vi "Set Scan Settings.vi"(10 "Test Settings":T1 {"Load Cell Sensitivity" format="%.6f"}, 11 "Model in":refnum<class "Model.lvclass">) -> (3 "Model out":refnum<class "Model.lvclass">)   [LabVIEW 2016]
uses:
  Model.lvclass
  Typedefs/TestSettings.ctl
  Typedefs/HPMT_Typedefs.lvlib
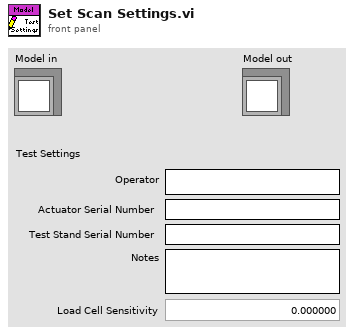
[diagram p1: front panel]
types:
  T1 = typedef "HPMT_Typedefs.lvlib/TestSettings.ctl" = cluster{"Operator":string, "Actuator Serial Number":string, "Test Stand Serial Number":string, "Notes":string, "Load Cell Sensitivity":dbl}
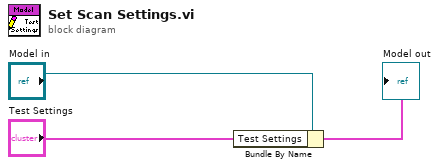
[diagram p0: block diagram]
diagram:
  n1 = Bundle By Name(cluster="Model in", "Test Settings"="Test Settings") -> (→"Model out":cluster{})
